vi "MGI Coerce Panel Bounds to Viewable Area.vi"(8 "Error In":errorcluster, 11 "Panel Bounds In":T1) -> (0 "Error Out":errorcluster, 3 "Panel Bounds Out":T1)   [LabVIEW 2016]
doc: "Coerce the specified panel bounds to fit on screen. If at least a 50 pixel square of the top left or top right rectangle appear on one of the monitors, then the original panel bounds is output. Otherwise, the panel bounds are changed to appear on the primary monitor.\n\nAuthored by Shawn Walpole\nsupport@mooregoodideas.com\nwww.mooregoodideas.com\n\nCopyright (c) 2010, Moore Good Ideas, Inc.\n\nAll rights reserved.\n\nRedistribution and use in source and binary forms, with or without modification, are permitted provided that the following conditions are met:\n\n * Redistributions of source code must retain the above copyright notice, this list of conditions and the following disclaimer.\n * Redistributions in binary form must reproduce the above copyright notice, this list of conditions and the following disclaimer in the documentation and/or other materials provided with the distribution.\n * Neither the name of Moore Good Ideas, Inc. nor the names of its contributors may be used to endorse or promote products derived from this software without specific prior written permission.\n\nTHIS SOFTWARE IS PROVIDED BY THE COPYRIGHT HOLDERS AND CONTRIBUTORS \"AS IS\" AND ANY EXPRESS OR IMPLIED WARRANTIES, INCLUDING, BUT NOT LIMITED TO, THE IMPLIED WARRANTIES OF MERCHANTABILITY AND FITNESS FOR A PARTICULAR PURPOSE ARE DISCLAIMED. IN NO EVENT SHALL THE COPYRIGHT OWNER OR CONTRIBUTORS BE LIABLE FOR ANY DIRECT, INDIRECT, INCIDENTAL, SPECIAL, EXEMPLARY, OR CONSEQUENTIAL DAMAGES (INCLUDING, BUT NOT LIMITED TO, PROCUREMENT OF SUBSTITUTE GOODS OR SERVICES; LOSS OF USE, DATA, OR PROFITS; OR BUSINESS INTERRUPTION) HOWEVER CAUSED AND ON ANY THEORY OF LIABILITY, WHETHER IN CONTRACT, STRICT LIABILITY, OR TORT (INCLUDING NEGLIGENCE OR OTHERWISE) ARISING IN ANY WAY OUT OF THE USE OF THIS SOFTWARE, EVEN IF ADVISED OF THE POSSIBILITY OF SUCH DAMAGE."
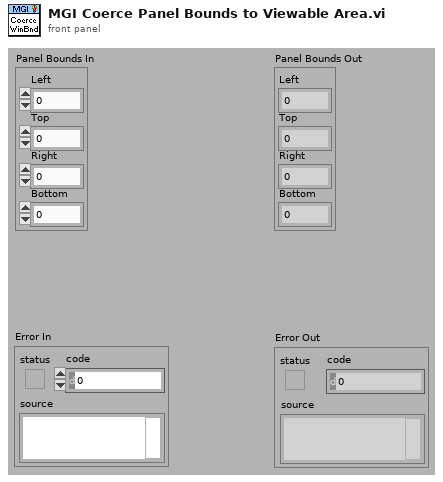
[diagram p1: front panel]
types:
  T1 = cluster{"Left":i16, "Top":i16, "Right":i16, "Bottom":i16}
  T2 = cluster{"left":i16, "top":i16, "right":i16, "bottom":i16}
  T3 = typedef "LVAllMonitorsDisplayTypeDef.ctl" = cluster{"Bounds":cluster{"Left":i16, "Top":i16, "Right":i16, "Bottom":i16}, "Depth":i16}[]
  T4 = typedef "LVRectTypeDef.ctl" = cluster{"Left":i16, "Top":i16, "Right":i16, "Bottom":i16}
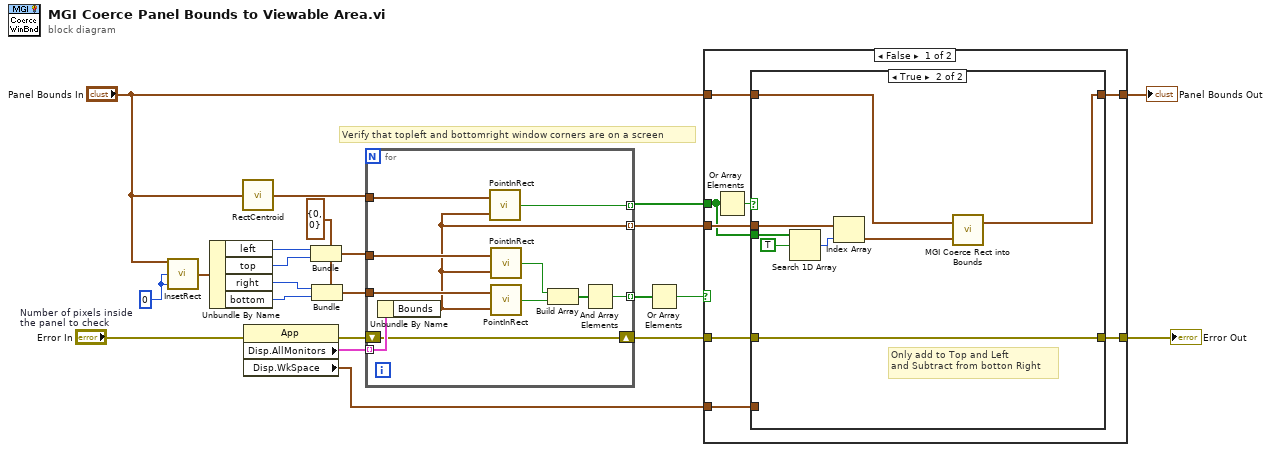
[diagram p0: block diagram]
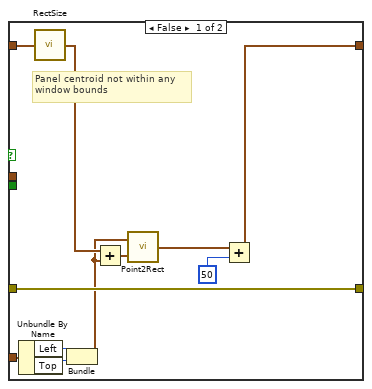
[diagram p2: hidden frame]
diagram:
  w9 = i16 0  # Number of pixels inside the panel to check
  w5 = cluster{"x":i16, "y":i16} {"x"=0, "y"=0} ("point")
  # "Verify that topleft and bottomright window corners are on a screen"
  n1 = call <vilib>:"InsetRect.vi"("dv"=w9, "dh"=w9, "rect"="Panel Bounds In") -> ("inset rect"=w17:T2)
  n2 = Unbundle By Name(w17) -> ("left"=w19:i16, "top"=w18:i16, "right"=w8:i16, "bottom"=w7:i16)
  n3 = call <vilib>:"RectCentroid.vi"("rect"="Panel Bounds In") -> ("point"=w3:cluster{"x":i16, "y":i16})
  n4 = property class="App"(error in="Error In") -> (error out=w20:errorcluster, "Disp.AllMonitors"=w22:T3, "Disp.WkSpace"=w10:T4)  [unwired: 1 in, 1 out]
  n5 = Bundle(cluster=w5, "x"=w19, "y"=w18) -> (w16:cluster{"x":i16, "y":i16})
  n6 = Bundle(cluster=w5, "x"=w8, "y"=w7) -> (w6:cluster{"x":i16, "y":i16})
  n7 = for {
    tunnel: w22 -> [w33] mode=indexing
    shift-right: [w31] -> w13
    shift-left: w20 -> [w31]
    tunnel: w16 -> [w32]
    tunnel: [w27] -> w15 mode=indexing
    tunnel: w6 -> [w26]
    tunnel: w3 -> [w25]
    tunnel: [w24] -> w2 mode=indexing
    tunnel: [w23] -> w1 mode=indexing
    n8 = Unbundle By Name(w33) -> ("Bounds"=w23:T1)
    n9 = call <vilib>:"PointInRect.vi"("rect"=w23, "point"=w25) -> ("pt in rect"=w24:bool)
    n10 = call <vilib>:"PointInRect.vi"("rect"=w23, "point"=w32) -> ("pt in rect"=w30:bool)
    n11 = call <vilib>:"PointInRect.vi"("rect"=w23, "point"=w26) -> ("pt in rect"=w29:bool)
    n12 = Build Array(w30, w29) -> (w28:bool[])
    n13 = And Array Elements(Boolean array=w28) -> (logical AND=w27:bool)
  }
  n14 = Or Array Elements(Boolean array=w15) -> (logical OR=w14:bool)
  n15 = case shown="False" w14 {
    tunnel: w13 -> [w36 w62]
    tunnel: [w35 w62] -> w12
    tunnel: "Panel Bounds In" -> [w40 w61]
    tunnel: [w39 w61] -> w11
    tunnel: w10 -> [w41 _]
    tunnel: w2 -> [w34 _]
    tunnel: w1 -> [w37 _]
    frame False {
      n16 = Or Array Elements(Boolean array=w34) -> (logical OR=w38:bool)
      n17 = case shown="True" w38 {
        tunnel: w41 -> [w52 _]
        tunnel: w40 -> [w48 w55]
        tunnel: [w46 w53] -> w39
        tunnel: w37 -> [_ w57]
        tunnel: w36 -> [w45 w60]
        tunnel: [w45 w60] -> w35
        tunnel: w34 -> [_ w59]
        frame False {
          # "Panel centroid not within any\nwindow bounds"
          n18 = Unbundle By Name(w52) -> ("Left"=w51:i16, "Top"=w50:i16)
          n19 = call <vilib>:"RectSize.vi"("rect"=w48) -> ("point"=w44:cluster{"x":i16, "y":i16})
          n20 = Bundle("Left"=w51, "Top"=w50) -> (w42:cluster{"Left":i16, "Top":i16})  [unwired: 1 in]
          n21 = Add(x=w44, y=w42) -> (x+y=w43:cluster{i16, i16})
          n22 = call <vilib>:"Point2Rect.vi"("point b"=w43, "point a"=w42) -> ("rect"=w47:T2)
          n23 = Add(x=w47, y=i16 50) -> (x+y=w46:T2)
        }
        frame True {
          # "Only add to Top and Left\nand Subtract from botton Right"
          n24 = Search 1D Array(1D array=w59, element=TRUE) -> (index of element=w56:i32)  [unwired: 1 in]
          n25 = Index Array(array=w57, index=w56) -> (element=w54:T1)
          n26 = call <userlib>:"MGI Coerce Rect into Bounds.vi"("Bounds"=w54, "Rect"=w55) -> ("Coerced Rect"=w53:T1)  [unwired: 1 out]
        }
      }
    }
    frame True {
    }
  }
  "Error Out" <- w12
  "Panel Bounds Out" <- w11
